vi "motor temp.vi"(8 "error in (no error)":errorcluster, 9 "DELAY (ms) in":u32, 10 "Dup Controller # in":string, 11 "VISA Refnum in":refnum<visa-resource-name>) -> (0 "error out":errorcluster, 1 "Temperature":dbl, 2 "Dup Controller # out":string, 3 "VISA Refnum out":refnum<visa-resource-name>)   [LabVIEW 2014]
doc: "gives temperature of the motor/controller"
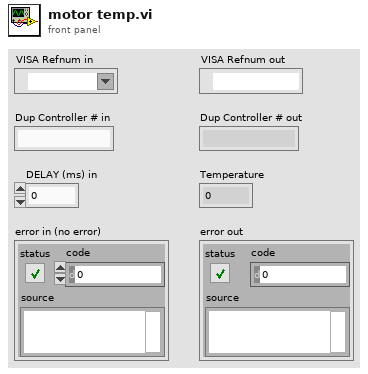
[diagram p1: front panel]
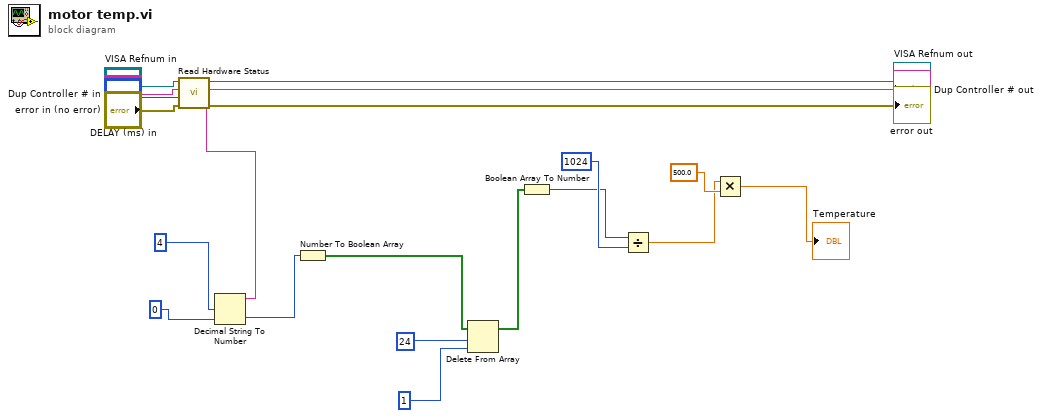
[diagram p0: block diagram]
diagram:
  n1 = call <userlib>:"Read Hardware Status.vi"("error in (no error)"="error in (no error)", "Delay (ms)"="DELAY (ms) in", "Controller #"="Dup Controller # in", "VISA Handle"="VISA Refnum in") -> ("error out"=→"error out":errorcluster, "Response"=w11:string, "Dup Controller #"=→"Dup Controller # out":string, "Dup VISA Handle"=→"VISA Refnum out":refnum<visa-resource-name>)  [unwired: 2 out]
  n2 = Decimal String To Number(string=w11, offset=4, default (0L)=0 ("default (0 I32)")) -> (number=w9:i32)  [unwired: 1 out]
  n3 = Number To Boolean Array(number=w9) -> (Boolean array=w1:bool[])
  n4 = Delete From Array(array=w1, length=24, index=1) -> (array with subset deleted=w10:bool[])  [unwired: 1 out]
  n5 = Boolean Array To Number(Boolean array=w10) -> (number=w3:u32)
  n6 = Divide(x=w3, y=u32 1024) -> (x/y=w5:dbl)
  n7 = Multiply(x=w5, y=500.0) -> (x*y=→"Temperature":dbl)
